vi "Read connection.vi"(8 "error in (no error)":errorcluster, 11 "RP Communicator in":refnum<class "RP Communicator VISA.lvclass">) -> (0 "error out":errorcluster, 2 "connection":refnum<visa-resource-name>, 3 "RP Communicator out":refnum<class "RP Communicator VISA.lvclass">)   [LabVIEW 2016, in "RP Communicator VISA.lvclass"]
uses:
  RP Communicator VISA.lvclass
  RP Communicator VISA.lvclass/RP Communicator VISA.ctl
panel:
  out "NaN/Path/Refnum?":bool
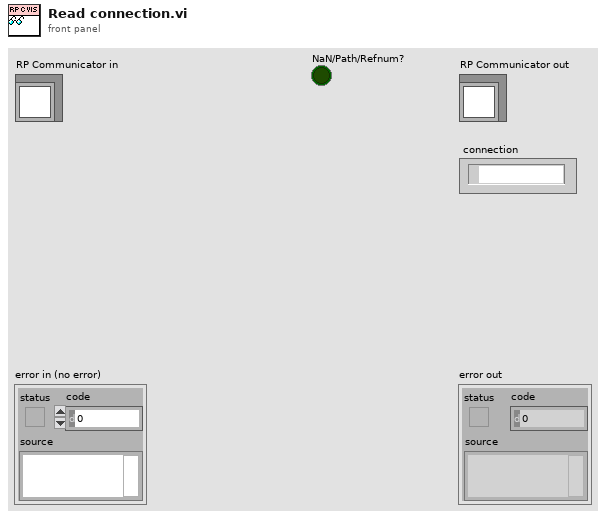
[diagram p1: front panel]
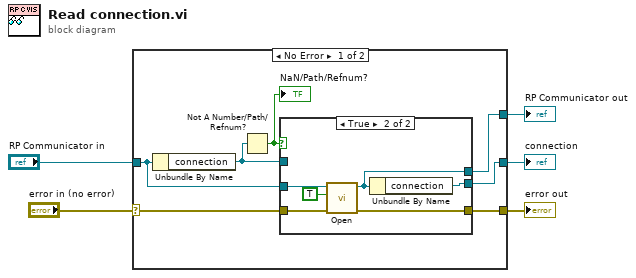
[diagram p0: block diagram]
diagram:
  n1 = case shown="No Error" "error in (no error)" {
    selector: "error in (no error)" -> [w9 w22]
    tunnel: [w8 w22] -> w4
    tunnel: [w10 w23] -> w2
    tunnel: "RP Communicator in" -> [w11 w23]
    tunnel: [w6 _] -> w1
    frame No Error {
      n2 = Unbundle By Name(w11) -> ("connection"=w7:refnum<visa-resource-name>)
      n3 = Not A Number/Path/Refnum?(number/path/refnum=w7) -> (NaN/Path/Refnum?=w12:bool)
      "NaN/Path/Refnum?" <- w12
      n4 = case shown="True" w12 {
        tunnel: w11 -> [w15 w19]
        tunnel: [w15 w18] -> w10
        tunnel: w9 -> [w14 w21]
        tunnel: [w14 w20] -> w8
        tunnel: w7 -> [w13 _]
        tunnel: [w13 w17] -> w6
        frame False {
        }
        frame True {
          n5 = call-dynamic "Open.vi"("error in (no error)"=w21, "Send \"Connect client\""=TRUE ("Send \"Connect client\""), "RP Communicator in"=w19) -> ("error out"=w20:errorcluster, "RP Communicator out"=w18:refnum<class "RP Communicator VISA.lvclass">)  [unwired: 7 in]
          n6 = Unbundle By Name(w18) -> ("connection"=w17:refnum<visa-resource-name>)
        }
      }
    }
    frame Error {
    }
  }
  "error out" <- w4
  "RP Communicator out" <- w2
  "connection" <- w1
